vi "WriteSingleFrame.vi"(4 "ArbitrationId":u32 format="%08x", 5 "DataLength":u8, 8 "error in":errorcluster, 9 "IsRemote":u8, 10 "Data":u8[](array[numeric]) format="%02x", 11 "CanHandleIn":T1) -> (0 "error out":errorcluster, 3 "CanHandleOut":T1)   [LabVIEW 2011, in "Konvolucio MCAN120803.lvlib"]
uses:
  <instrlib>/Konvolucio MCAN120803/Konvolucio MCAN120803.lvlib
  <instrlib>/Konvolucio MCAN120803/Types/CanHandleType.ctl
  C:/Program Files/National Instruments/LabVIEW 2011/instr.lib/Konvolucio MCAN120803/Private/Konvolucio.MCAN120803.API.dll
  Private/Konvolucio.MCAN120803.API.dll
  <instrlib>/Konvolucio MCAN120803/Types/MessageType.ctl
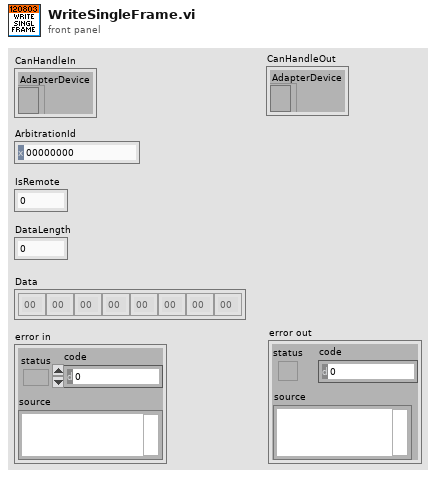
[diagram p1: front panel]
types:
  T1 = typedef "Konvolucio MCAN120803.lvlib/CanHandleType.ctl" = cluster{"AdapterDevice":refnum<k24>}
  T2 = typedef "Konvolucio MCAN120803.lvlib/MessageType.ctl" = cluster{"TimeStamp":timestamp, "ArbitrationId":u32, "IsRemote":u8, "DataLength":u8, "Data":u8[]}
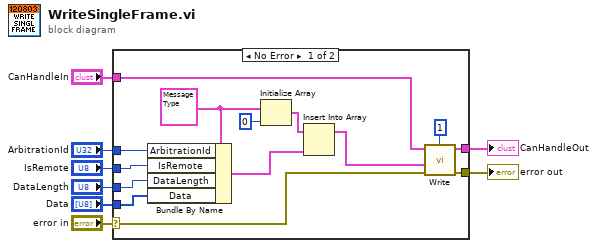
[diagram p0: block diagram]
diagram:
  n1 = case shown="No Error" "error in" {
    selector: "error in" -> [w9 w24]
    tunnel: "ArbitrationId" -> [w16 _]
    tunnel: "DataLength" -> [w15 _]
    tunnel: "IsRemote" -> [w14 _]
    tunnel: "Data" -> [w13 _]
    tunnel: "CanHandleIn" -> [w12 w23]
    tunnel: [w11 w23] -> w3
    tunnel: [w10 w24] -> w2
    frame No Error {
      w18 = T2 {"TimeStamp"=timestamp(0 s since 1904-01-01), "ArbitrationId"=0, "IsRemote"=0, "DataLength"=0, "Data"=[]}
      n2 = Bundle By Name(cluster=w18, "ArbitrationId"=w16, "IsRemote"=w14, "DataLength"=w15, "Data"=w13) -> (w17:T2)
      n3 = Initialize Array(w18, 0 ("dimension size")) -> (w20:T2[])
      n4 = Insert Into Array(array=w20, new element=w17) -> (w19:T2[])  [unwired: 1 in]
      n5 = call <instrlib>:"Write.vi"("error in"=w9, "Messages"=w19, "Number to Write"=1, "CanHandleIn"=w12) -> ("error out"=w10:errorcluster, "CanHandleOut"=w11:T1)  [unwired: 4 in]
    }
    frame Error {
    }
  }
  "CanHandleOut" <- w3
  "error out" <- w2
